vi "SV Open Excel.vi"(1 "error in (no error)":errorcluster) -> (0 "error out":errorcluster, 2 "Refnum Cluster":T1)   [LabVIEW 2010]
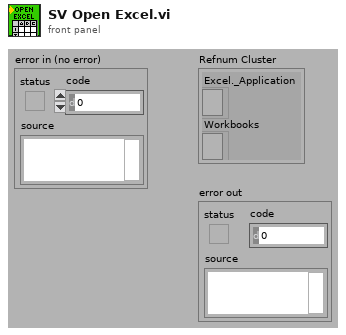
[diagram p1: front panel]
types:
  T1 = cluster{"Excel._Application":refnum<k7>, "Workbooks":refnum<k7>}
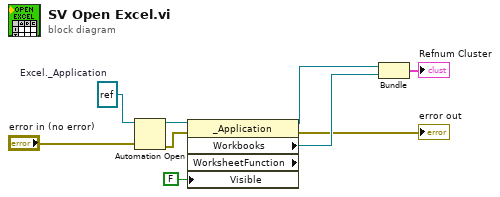
[diagram p0: block diagram]
diagram:
  w4 = refnum<k7> refnum  # Excel._Application
  n1 = Automation Open(error in (no error)="error in (no error)", Automation Refnum=w4) -> (Automation Refnum=w8:refnum<k7>, error out=w3:errorcluster)  [unwired: 2 in]
  n2 = property class="_Application" props=["Workbooks", "WorksheetFunction", "Visible"](reference=w8, error in=w3, "Visible"=FALSE) -> (reference out=w5:refnum<k7>, error out=→"error out":errorcluster, "Workbooks"=w6:refnum<k7>)  [unwired: 1 out]
  n3 = Bundle("Excel._Application"=w5, "Workbooks"=w6) -> (→"Refnum Cluster":T1)  [unwired: 1 in]
